vi "ReadWriteClassAttribute.vi"(5 "error in (no error)":errorcluster) -> (19 "error out":errorcluster)   [LabVIEW 2017, in "G#MethodTemplates.lvclass"]
uses:
  <vilib>/addons/_AddQ/G#Templates/G#MethodTemplates/G#MethodTemplates.lvclass
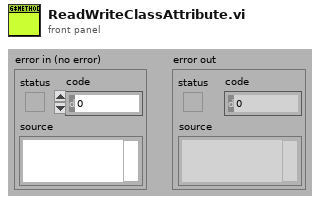
[diagram p1: front panel]
types:
  T1 = typedef "G#MethodTemplates.lvclass/ClassAttributesRef.ctl" = refnum<data-value>
  T2 = typedef "G#MethodTemplates.lvclass/ClassAttributes.ctl" = cluster{"Dummy":bool}
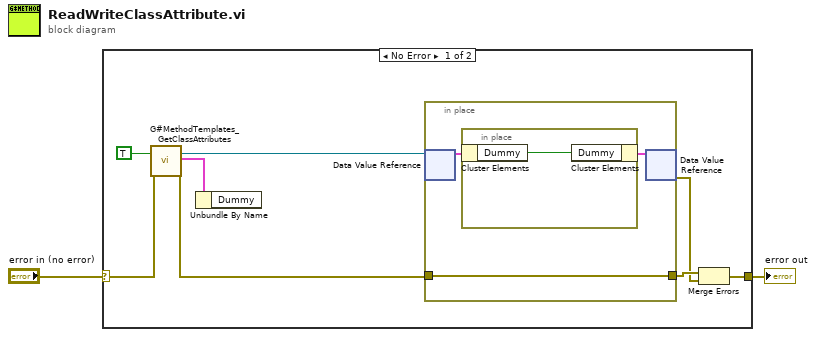
[diagram p0: block diagram]
diagram:
  n1 = case shown="No Error" "error in (no error)" {
    selector: "error in (no error)" -> [w10 w15]
    tunnel: [w7 w15] -> w1
    frame No Error {
      n2 = call <vilib>:"G#MethodTemplates_GetClassAttributes.vi"("return data? (T)"=TRUE ("return data"), "error in (no error)"=w10) -> ("class attributes ref"=w8:T1, "class attributes"=w5:T2, "error out"=w9:errorcluster)  [unwired: 14 in, 1 out]
      n3 = Unbundle By Name(w5) -> ()  [unwired: 1 out]
      n4 = in-place {
        in-place-border: w9 -> [w11]
        in-place-border: [w11] -> w4
        n5 = in-place-dvr #1(w8) -> (w12:T2)  [unwired: 1 out]
        n6 = in-place {
          n7 = in-place-cluster #2(w12) -> ("Dummy"=w14:bool)
          n8 = in-place-cluster #2("Dummy"=w14) -> (w13:T2)
        }
        n9 = in-place-dvr #1(w13) -> (w3:errorcluster)  [unwired: 1 out]
      }
      n10 = Merge Errors(w4, w3) -> (w7:errorcluster)
    }
    frame Error {
    }
  }
  "error out" <- w1
